vi "Dialog Box.vi"(8 "error in (no error)":errorcluster, 11 "SubPanel in":refnum<class "SubPanel.lvclass">) -> (0 "error out":errorcluster, 1 "timed out?":bool, 2 "Selection":string, 3 "SubPanel out":refnum<class "SubPanel.lvclass">)   [LabVIEW 2012, in "SubPanel.lvlib" / "SubPanel.lvclass"]
doc: "This VI contains the code for the dialog box.\nOverride this VI to provide more functionality or to create your own application-specific dialog box."
uses:
  SubPanel.lvclass
  <vilib>/Utility/miscctls.llb/LVBoundsTypeDef.ctl
  <vilib>/Utility/miscctls.llb/LVPositionTypeDef.ctl
  SubPanel.lvclass/SubPanel.ctl
  Fading/_Fade In(I32).vi
panel:
  out "String":string
  out "Picture":picture
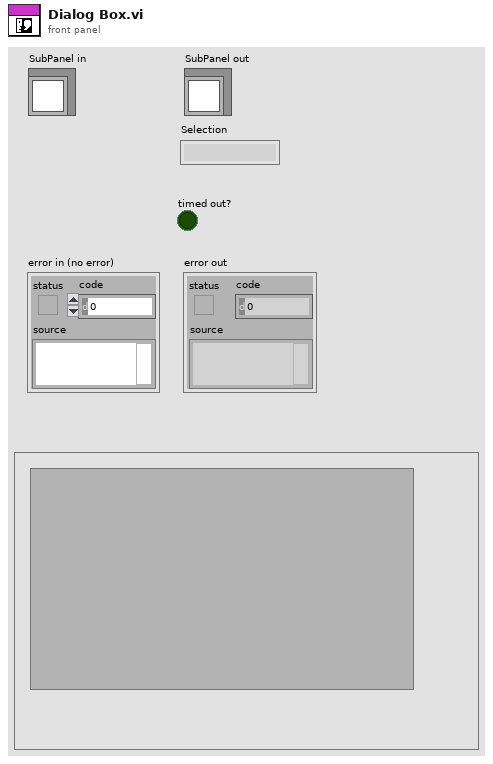
[diagram p1: front panel]
types:
  T1 = typedef "LVPositionTypeDef.ctl" = cluster{"Left":i32, "Top":i32}
  T2 = typedef "LVBoundsTypeDef.ctl" = cluster{"Width":u32, "Height":u32}
  T3 = typedef "imagedata.ctl" = cluster{"image type":i32, "image depth":i32, "image":u8[], "mask":u8[], "colors":u32[], "Rectangle":cluster{"left":i16, "top":i16, "right":i16, "bottom":i16}}
  T4 = cluster{"left":i16, "top":i16, "right":i16, "bottom":i16}
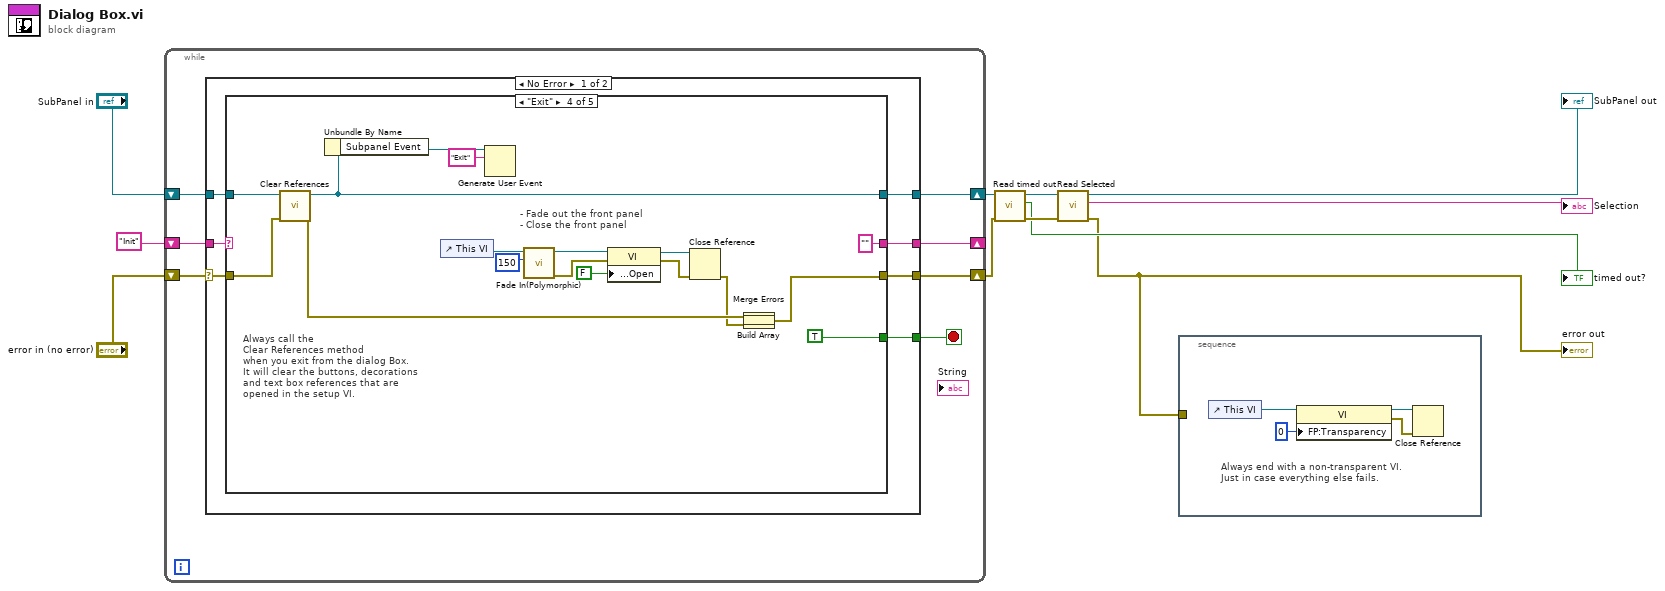
[diagram p0: block diagram]
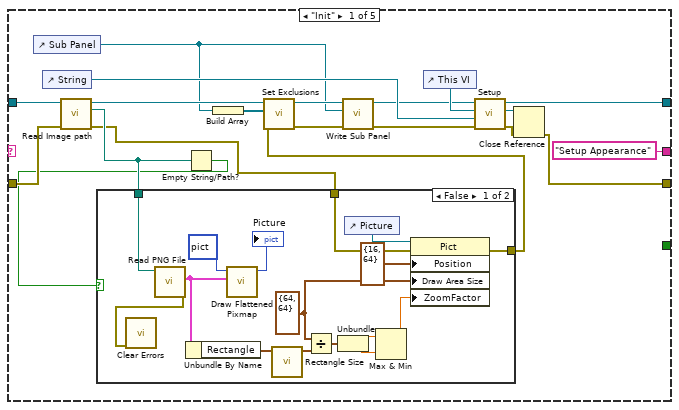
[diagram p2: hidden frame]
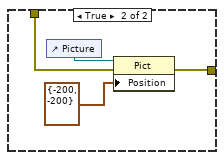
[diagram p3: hidden frame]
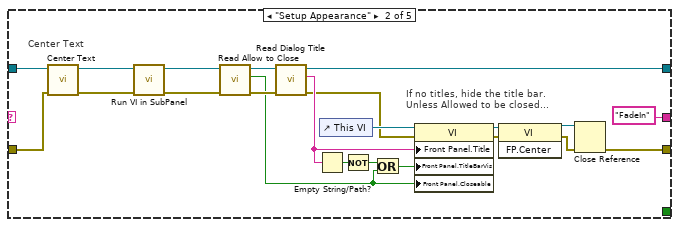
[diagram p4: hidden frame]
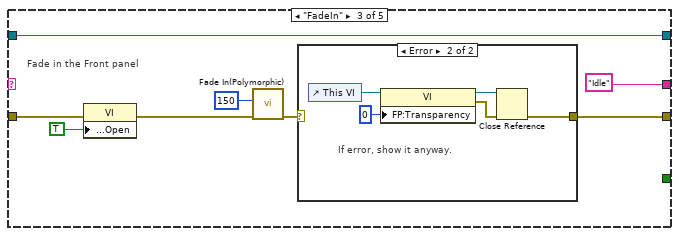
[diagram p5: hidden frame]
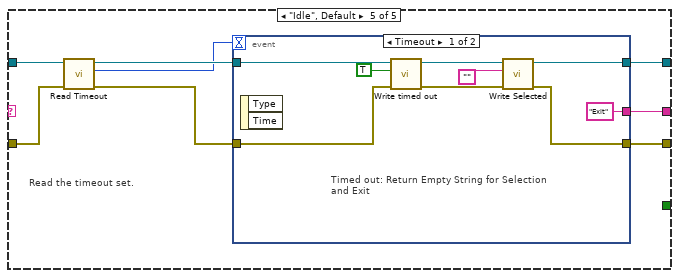
[diagram p7: hidden frame]
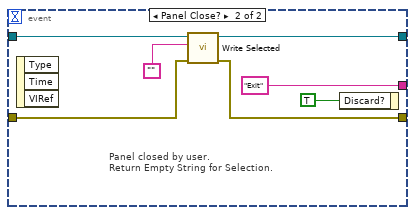
[diagram p8: hidden frame]
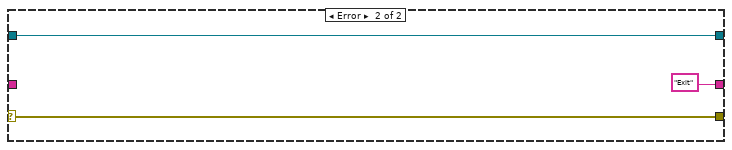
[diagram p9: hidden frame]
diagram:
  n1 = while {
    shift-right: [w14] -> _
    shift-left: "Init" -> [w15]
    shift-right: [w18] -> w10
    shift-left: "SubPanel in" -> [w17]
    shift-right: [w16] -> w9
    shift-left: "error in (no error)" -> [w12]
    stop <- w13 stop-if-true
    n2 = case shown="No Error" w12 {
      selector: w12 -> [w19 w144]
      tunnel: [w25 w146] -> w18
      tunnel: w17 -> [w24 w146]
      tunnel: [w23 w144] -> w16
      tunnel: w15 -> [w22 _]
      tunnel: [w21 "Exit"] -> w14
      tunnel: [w20 _] -> w13
      frame No Error {
        n3 = case shown="\"Exit\"" w22 {
          tunnel: [w43 w78 w95 w104 w127] -> w25
          tunnel: w24 -> [w35 w76 w95 w110 w124]
          tunnel: [w40 w79 w91 w106 w126] -> w23
          tunnel: w19 -> [w39 w75 w90 w109 w121]
          tunnel: ["Setup Appearance" "FadeIn" "Idle" "" w125] -> w21
          tunnel: [_ _ _ TRUE _] -> w20
          frame "Init" {
            n4 = control-ref of="Sub Panel"() -> (w29:refnum<vi>)
            n5 = control-ref of="String"() -> (w33:refnum<vi>)
            n6 = call-dynamic "Read Image path.vi"("error in (no error)"=w39, "MessageBox.lvclass in"=w35) -> ("error out"=w28:errorcluster, "Image path"=w38:path, "MessageBox.lvclass out"=w36:refnum<class "SubPanel.lvclass">)  [unwired: 7 out]
            n7 = Empty String/Path?(string/path=w38) -> (empty?=w37:bool)
            n8 = case shown="False" w37 {
              tunnel: w38 -> [w52 _]
              tunnel: [w50 w65] -> w27
              tunnel: w28 -> [w49 w64]
              frame False {
                w61 = T2 {"Width"=64, "Height"=64} ("Draw Area Size")
                n9 = call <vilib>:"Read PNG File.vi"("path to PNG file"=w52) -> ("error out"=w51:errorcluster, "image data"=w54:T3)  [unwired: 1 in, 8 out]
                n10 = call <vilib>:"Clear Errors.vi"("error in (no error)"=w51) -> ()  [unwired: 7 out]
                n11 = Unbundle By Name(w54) -> ("Rectangle"=w55:T4)
                n12 = call <vilib>:"Draw Flattened Pixmap.vi"("image data"=w54, "picture"=picture data[5B]) -> ("new picture"=→"Picture":picture)  [unwired: 7 out]
                n13 = call "Rectangle Size.vi"("Rectangle"=w55) -> ("Rect Size"=w60:cluster{"width":i32, "height":i32})  [unwired: 10 out]
                n14 = Divide(x=w61, y=w60) -> (x/y=w56:cluster{dbl, dbl})
                n15 = Unbundle(w56) -> (w57:dbl, w58:dbl)
                n16 = control-ref of="Picture"() -> (w46:refnum<vi>)
                n17 = Max & Min(x=w57, y=w58) -> (max(x,y)=w59:dbl)  [unwired: 1 out]
                n18 = property class="Pict"(reference=w46, error in=w49, "Position"=T1 {"Left"=16, "Top"=64}, "Draw Area Size"=w61, "ZoomFactor"=w59) -> (error out=w50:errorcluster)  [unwired: 1 out]
              }
              frame True {
                n19 = control-ref of="Picture"() -> (w62:refnum<vi>)
                n20 = property class="Pict"(reference=w62, error in=w64, "Position"=T1 {"Left"=-200, "Top"=-200}) -> (error out=w65:errorcluster)  [unwired: 1 out]
              }
            }
            n21 = Build Array(w29) -> (w34:refnum<vi>[])
            n22 = call-dynamic "Set Exclusions.vi"("error in (no error)"=w27, "Exclusions"=w34, "Dialog in"=w36) -> ("error out"=w32:errorcluster, "Dialog out"=w31:refnum<class "SubPanel.lvclass">)  [unwired: 7 out]
            n23 = call-dynamic "Write Sub Panel.vi"("error in (no error)"=w32, "Sub Panel"=w29, "SubPanel.lvclass in"=w31) -> ("error out"=w26:errorcluster, "SubPanel.lvclass out"=w30:refnum<class "SubPanel.lvclass">)  [unwired: 7 out]
            n24 = control-ref of="This VI"() -> (w44:refnum<vi>)
            n25 = call-dynamic "Setup.vi"("error in (no error)"=w26, "Str Refnum"=w33, "VI Reference"=w44, "Dialog in"=w30) -> ("error out"=w41:errorcluster, "VI reference (dup)"=w42:refnum<vi>, "Dialog out"=w43:refnum<class "SubPanel.lvclass">)  [unwired: 5 out]
            n26 = Close Reference(reference=w42, error in (no error)=w41) -> (error out=w40:errorcluster)
          }
          frame "Setup Appearance" {
            # "Center Text"
            # "If no titles, hide the title bar.\nUnless Allowed to be closed..."
            n27 = call-dynamic "Center Text.vi"("error in (no error)"=w75, "SubPanel in"=w76) -> ("error out"=w66:errorcluster, "SubPanel out"=w69:refnum<class "SubPanel.lvclass">)  [unwired: 8 out]
            n28 = call-dynamic "Run VI in SubPanel.vi"("error in (no error)"=w66, "SubPanel in"=w69) -> ("error out"=w67:errorcluster, "SubPanel out"=w68:refnum<class "SubPanel.lvclass">)  [unwired: 8 out]
            n29 = call-dynamic "Read Allow to Close.vi"("error in (no error)"=w67, "Dialog.lvclass in"=w68) -> ("error out"=w73:errorcluster, "Allow to close?"=w70:bool, "Dialog.lvclass out"=w74:refnum<class "SubPanel.lvclass">)  [unwired: 7 out]
            n30 = call-dynamic "Read Dialog Title.vi"("error in (no error)"=w73, "Dialog in"=w74) -> ("error out"=w77:errorcluster, "Dialog Title"=w82:string, "Dialog out"=w78:refnum<class "SubPanel.lvclass">)  [unwired: 7 out]
            n31 = Empty String/Path?(string/path=w82) -> (empty?=w85:bool)
            n32 = control-ref of="This VI"() -> (w86:refnum<vi>)
            n33 = Not(x=w85) -> (.not. x?=w72:bool)
            n34 = Or(x=w72, y=w70) -> (x .or. y?=w71:bool)
            n35 = property class="VI"(reference=w86, error in=w77, "Front Panel.Title"=w82, "Front Panel.TitleBarVis"=w71, "Front Panel.Closeable"=w70) -> (reference out=w84:refnum<vi>, error out=w83:errorcluster)
            n36 = invoke class="VI" method="FP.Center"(reference=w84, error in=w83) -> (reference out=w81:refnum<vi>, error out=w80:errorcluster)  [unwired: 1 in, 1 out]
            n37 = Close Reference(reference=w81, error in (no error)=w80) -> (error out=w79:errorcluster)
          }
          frame "FadeIn" {
            # "Fade in the Front panel"
            n38 = property class="VI"(error in=w90, "Front Panel.Open"=TRUE ("Front Panel Window:Open")) -> (error out=w89:errorcluster)  [unwired: 1 in, 1 out]
            n39 = call-poly "Fade In(Polymorphic).vi"("error in"=w89, "Fade time (ms)"=150) -> ("error out"=w92:errorcluster)  [unwired: 2 in, 7 out]
            n40 = case shown="Error" w92 {
              selector: w92 -> [w96 _]
              tunnel: [w96 w97] -> w91
              frame No Error {
              }
              frame Error {
                # "If error, show it anyway."
                n41 = control-ref of="This VI"() -> (w99:refnum<vi>)
                n42 = property class="VI"(reference=w99, "FP:Transparency"=u8 0 ("Front Panel Window:Transparency")) -> (reference out=w100:refnum<vi>, error out=w101:errorcluster)  [unwired: 1 in]
                n43 = Close Reference(reference=w100, error in (no error)=w101) -> (error out=w97:errorcluster)
              }
            }
          }
          frame "Exit" {
            # "Always call the\nClear References method\nwhen you exit from the dialog Box.\nIt will clear the buttons, decorations\nand text box references that are \nopened in the setup VI."
            # "- Fade out the front panel\n- Close the front panel"
            n44 = call-dynamic "Clear References.vi"("error in (no error)"=w109, "Dialog in"=w110) -> ("error out"=w108:errorcluster, "Dialog out"=w104:refnum<class "SubPanel.lvclass">)  [unwired: 8 out]
            n45 = Unbundle By Name(w104) -> ("Subpanel Event"=w103:refnum<user-event>)
            n46 = control-ref of="This VI"() -> (w116:refnum<vi>)
            n47 = Generate User Event(user event=w103, event data cluster="Exit" ("event data")) -> ()  [unwired: 1 in, 2 out]
            n48 = call-poly "Fade In(Polymorphic).vi"("Fade time (ms)"=150, "VI Reference (calling VI)"=w116) -> ("error out"=w114:errorcluster, "dup VI Reference"=w115:refnum<vi>)  [unwired: 2 in, 6 out]
            n49 = property class="VI"(reference=w115, error in=w114, "Front Panel.Open"=FALSE ("Front Panel Window:Open")) -> (reference out=w112:refnum<vi>, error out=w111:errorcluster)
            n50 = Close Reference(reference=w112, error in (no error)=w111) -> (error out=w107:errorcluster)
            n51 = Build Array(w108, w107) -> (w105:errorcluster[])
            n52 = Merge Errors(w105) -> (w106:errorcluster)
          }
          frame "Idle", Default {
            # "Read the timeout set."
            n53 = call-dynamic "Read Timeout.vi"("error in (no error)"=w121, "Dialog.lvclass in"=w124) -> ("error out"=w120:errorcluster, "Timeout"=w122:i32, "Dialog.lvclass out"=w123:refnum<class "SubPanel.lvclass">)  [unwired: 7 out]
            n54 = event shown="[0] Timeout" {
              selector: _ -> [_ _]
              dyn-events: _ -> [_ _]
              timeout: w122 -> [_ _]
              tunnel: [w129 w139] -> w127
              tunnel: w123 -> [w135 w140]
              tunnel: [w130 w137] -> w126
              tunnel: w120 -> [w133 w138]
              tunnel: ["Exit" "Exit"] -> w125
              event Timeout {
                # "Timed out: Return Empty String for Selection\nand Exit"
                n55 = event-data() -> ()  [unwired: 3 out]
                n56 = call-dynamic "Write timed out.vi"("error in (no error)"=w133, "timed out?"=TRUE, "Dialog.lvclass in"=w135) -> ("error out"=w131:errorcluster, "Dialog.lvclass out"=w132:refnum<class "SubPanel.lvclass">)  [unwired: 7 out]
                n57 = call-dynamic "Write Selected.vi"("error in (no error)"=w131, "Selected"="", "Dialog.lvclass in"=w132) -> ("error out"=w130:errorcluster, "Dialog.lvclass out"=w129:refnum<class "SubPanel.lvclass">)  [unwired: 7 out]
              }
              event Panel Close? {
                # "Panel closed by user.\nReturn Empty String for Selection."
                n58 = event-data() -> ()  [unwired: 4 out]
                n59 = call-dynamic "Write Selected.vi"("error in (no error)"=w138, "Selected"="", "Dialog.lvclass in"=w140) -> ("error out"=w137:errorcluster, "Dialog.lvclass out"=w139:refnum<class "SubPanel.lvclass">)  [unwired: 7 out]
                n60 = event-data("Discard?"=TRUE) -> ()  [unwired: 1 in, 1 out]
              }
            }
          }
        }
      }
      frame Error {
      }
    }
  }
  n61 = call-dynamic "Read timed out.vi"("error in (no error)"=w9, "Dialog.lvclass in"=w10) -> ("error out"=w7:errorcluster, "timed out?"=→"timed out?":bool, "Dialog.lvclass out"=w8:refnum<class "SubPanel.lvclass">)  [unwired: 7 out]
  n62 = call-dynamic "Read Selected.vi"("error in (no error)"=w7, "Dialog.lvclass in"=w8) -> ("error out"=w3:errorcluster, "Selected"=→"Selection":string, "Dialog.lvclass out"=→"SubPanel out":refnum<class "SubPanel.lvclass">)  [unwired: 7 out]
  "error out" <- w3
  n63 = stacked-sequence {
    tunnel: w3 -> [_]
    frame #0 {
      # "Always end with a non-transparent VI.\nJust in case everything else fails."
      n64 = control-ref of="This VI"() -> (w149:refnum<vi>)
      n65 = property class="VI"(reference=w149, "FP:Transparency"=u8 0 ("Front Panel Window:Transparency")) -> (reference out=w148:refnum<vi>, error out=w147:errorcluster)  [unwired: 1 in]
      n66 = Close Reference(reference=w148, error in (no error)=w147) -> ()  [unwired: 1 out]
    }
  }
